vi "arreglos1.vi"() -> ()   [LabVIEW 2011]
panel:
  out "promedio":dbl
  out "Menor":dbl
  out "Mayor":dbl
  out "Suma":dbl
  out "Array":dbl[](array[numeric])
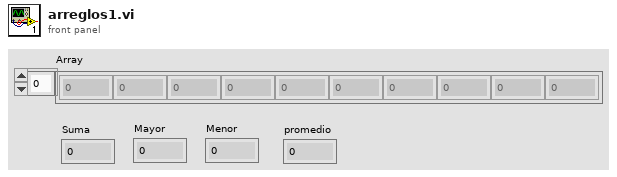
[diagram p1: front panel]
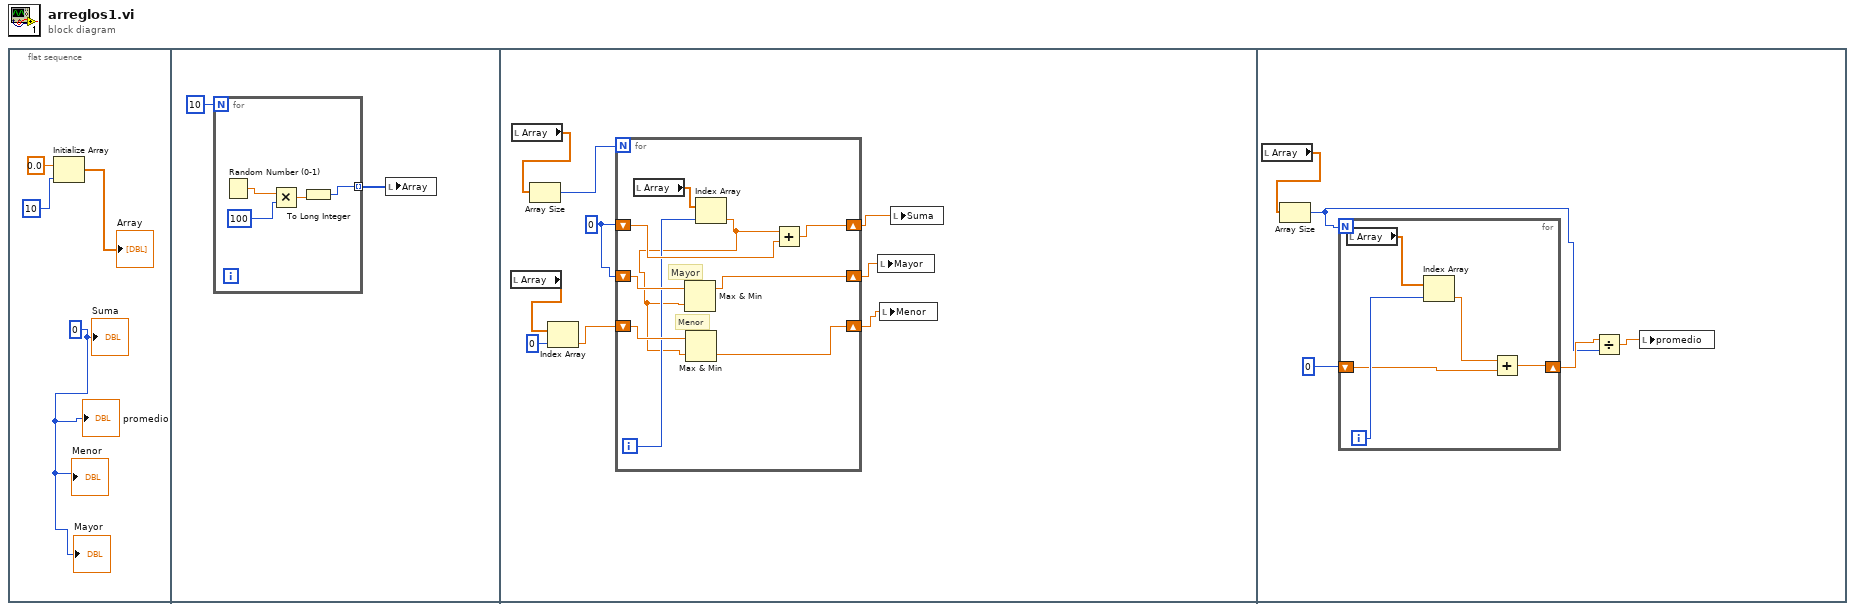
[diagram p0: block diagram]
diagram:
  n1 = flat-sequence {
    frame #0 {
      w1 = 0
      n2 = Initialize Array "Initialize Array"(0.0 ("element"), 10 ("dimension size")) -> (→"Array":dbl[])
      "Suma" <- w1
      "Mayor" <- w1
      "promedio" <- w1
      "Menor" <- w1
    }
    frame #1 {
      n3 = for {
        N: 10 -> [_]
        tunnel: [w7] -> w5 mode=indexing
        n4 = Random Number (0-1)() -> (number: 0 to 1=w9:dbl)
        n5 = Multiply(x=w9, y=100) -> (x*y=w8:dbl)
        n6 = To Long Integer(number=w8) -> (32bit integer=w7:i32)
      }
      n7 = local write "Array"(w5) -> ()
    }
    frame #2 {
      w17 = 0
      n8 = local read "Array"() -> (w16:dbl[])
      n9 = local read "Array"() -> (w19:dbl[])
      n10 = Array Size(array=w19) -> (size(s)=w11:i32)
      n11 = Index Array "Index Array"(array=w16, index=0) -> (element=w14:dbl)
      n12 = for {
        N: w11 -> [_]
        shift-right: [w27] -> w18
        shift-left: w17 -> [w26]
        shift-right: [w20] -> w13
        shift-left: w17 -> [w24]
        shift-right: [w21] -> w12
        shift-left: w14 -> [w25]
        i -> [w23]
        # "Menor"
        # "Mayor"
        n13 = local read "Array"() -> (w28:dbl[])
        n14 = Index Array "Index Array"(array=w28, index=w23) -> (element=w22:dbl)
        n15 = Max & Min(x=w24, y=w22) -> (max(x,y)=w20:dbl)  [unwired: 1 out]
        n16 = Max & Min(x=w25, y=w22) -> (min(x,y)=w21:dbl)  [unwired: 1 out]
        n17 = Add(x=w22, y=w26) -> (x+y=w27:dbl)
      }
      n18 = local write "Mayor"(w13) -> ()
      n19 = local write "Menor"(w12) -> ()
      n20 = local write "Suma"(w18) -> ()
    }
    frame #3 {
      n21 = local read "Array"() -> (w33:dbl[])
      n22 = Array Size(array=w33) -> (size(s)=w30:i32)
      n23 = for {
        N: w30 -> [_]
        shift-right: [w34] -> w31
        shift-left: 0 -> [w35]
        i -> [w37]
        n24 = local read "Array"() -> (w38:dbl[])
        n25 = Index Array "Index Array"(array=w38, index=w37) -> (element=w36:dbl)
        n26 = Add(x=w36, y=w35) -> (x+y=w34:dbl)
      }
      n27 = Divide(x=w31, y=w30) -> (x/y=w29:dbl)
      n28 = local write "promedio"(w29) -> ()
    }
  }
